vi "Stream Split Character Match RegExp Std Error.vi"(8 "error in (no error)":errorcluster, 11 "Bad Regex in":refnum<class "Bad Regex.lvclass">) -> (0 "error out":errorcluster, 2 "Stream Split Character Match RegExp Std Err":string)   [LabVIEW 2024, in "serenial.io-ase.test.lvlib" / "Bad Regex.lvclass"]
uses:
  Bad Regex.lvclass
  Bad Regex.lvclass/Bad Regex.ctl
  serenial.io-ase/configuration/configuration.lvclass
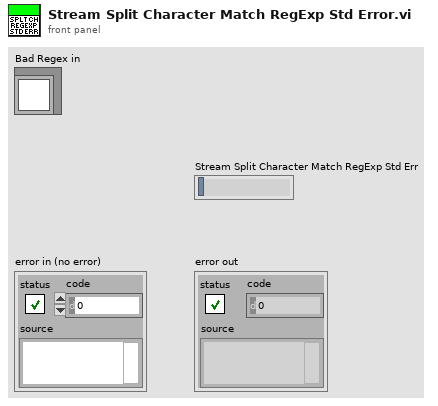
[diagram p1: front panel]
types:
  T1 = typedef "serenial.io-ase.test.lvlib/Bad Regex.lvclass/Bad Value.ctl" = enum16{"Out", "Err", "Both"}
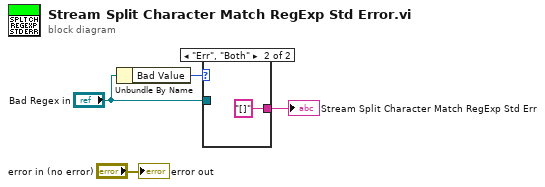
[diagram p0: block diagram]
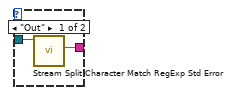
[diagram p2: hidden frame]
diagram:
  n1 = Unbundle By Name("Bad Regex in") -> ("Bad Value"=w3:T1)
  n2 = case shown="\"Err\", \"Both\"" w3 {
    tunnel: [w5 "[]"] -> w2
    tunnel: "Bad Regex in" -> [w6 _]
    frame "Out" {
      n3 = call-parent "Stream Split Character Match RegExp Std Error.vi"("configuration in"=w6) -> ("Stream Split Character Match RegExp Std Err"=w5:string)  [unwired: 9 in, 1 out]
    }
    frame "Err", "Both" {
    }
  }
  "Stream Split Character Match RegExp Std Err" <- w2
  "error out" <- "error in (no error)"
